vi "0630_Cinemática.vi"() -> ()   [LabVIEW 2017]
uses:
  <vilib>/robotics/Kinematics/Link/Joint Type.ctl
  <vilib>/robotics/Kinematics/RotateX.vi
  <vilib>/robotics/Kinematics/RotateY.vi
  <vilib>/robotics/Kinematics/RotateZ.vi
  <vilib>/Analysis/baseanly.llb/A x B.vi
  <vilib>/Analysis/baseanly.llb/Real A x B.vi
  <vilib>/robotics/Kinematics/Analytical/Initialize Generic Serial Arm.vi
  <vilib>/robotics/Kinematics/Robot/Inverse Kinematics (Point).vi
  <vilib>/picture/3D Picture Control/Object/Add Object (reference).vi
  <vilib>/robotics/Kinematics/Plotting/NI_Robotics_3DKinematics.lvlib
  <vilib>/robotics/Kinematics/Robot/NI_Robotics_Serial Robot Arm.lvclass
  <vilib>/robotics/Kinematics/Link/NI_Robotics_Link.lvclass
  <vilib>/robotics/Kinematics/Analytical/NI_Robotics_AnalyticKinematics.lvlib
  <vilib>/picture/3D Picture Control/NI_3D Picture Control.lvlib
  <vilib>/robotics/Kinematics/NI_Kinematics.lvlib
panel:
  in  "angles":cluster{"roll":dbl, "pitch":dbl, "yaw":dbl}
  in  "z":dbl
  in  "y":dbl
  in  "x":dbl
  out "error out":errorcluster
  out "3D Picture Control":refnum<vi>(3d-picture)
  in  "Stop Button":bool
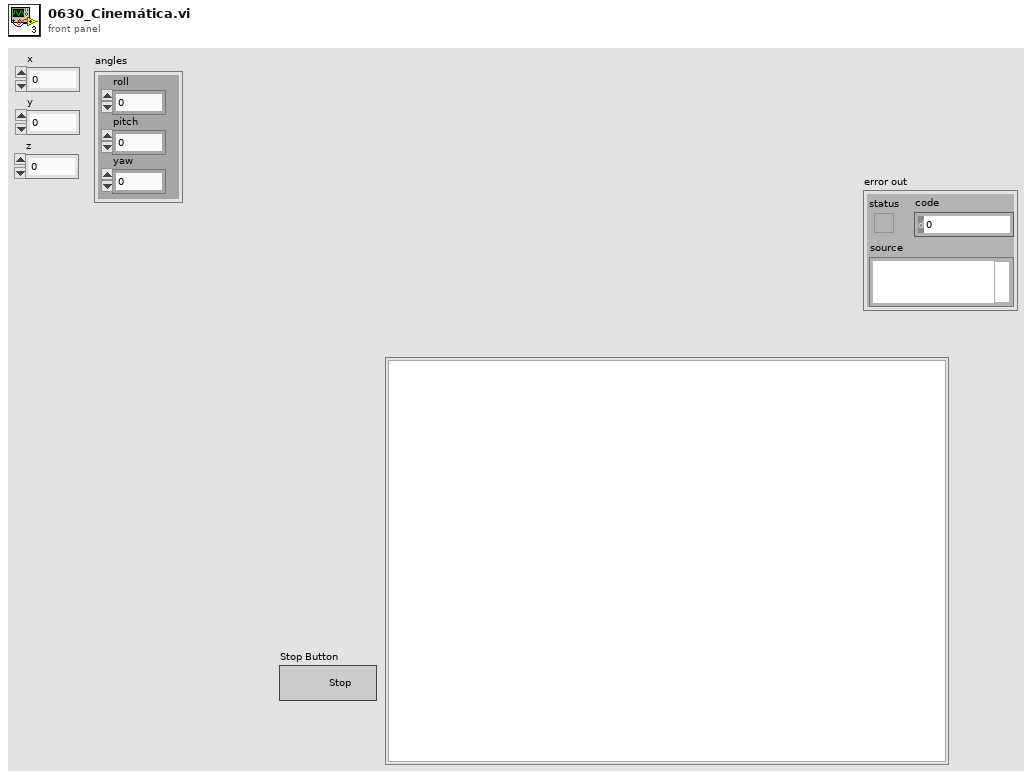
[diagram p1: front panel]
types:
  T1 = typedef "NI_Robotics_Link.lvclass/Joint Type.ctl" = enum16{"Revolute", "Prismatic"}
  T2 = cluster{"Twist Angle":dbl, "Length":dbl, "Rotation Angle":dbl, "Offset Distance":dbl, "Joint Type":T1, "Joint Coordinate Offset":dbl}[]
  T3 = typedef "NI_Matrix.lvlib/RealMatrix.ctl" = dbl[][]
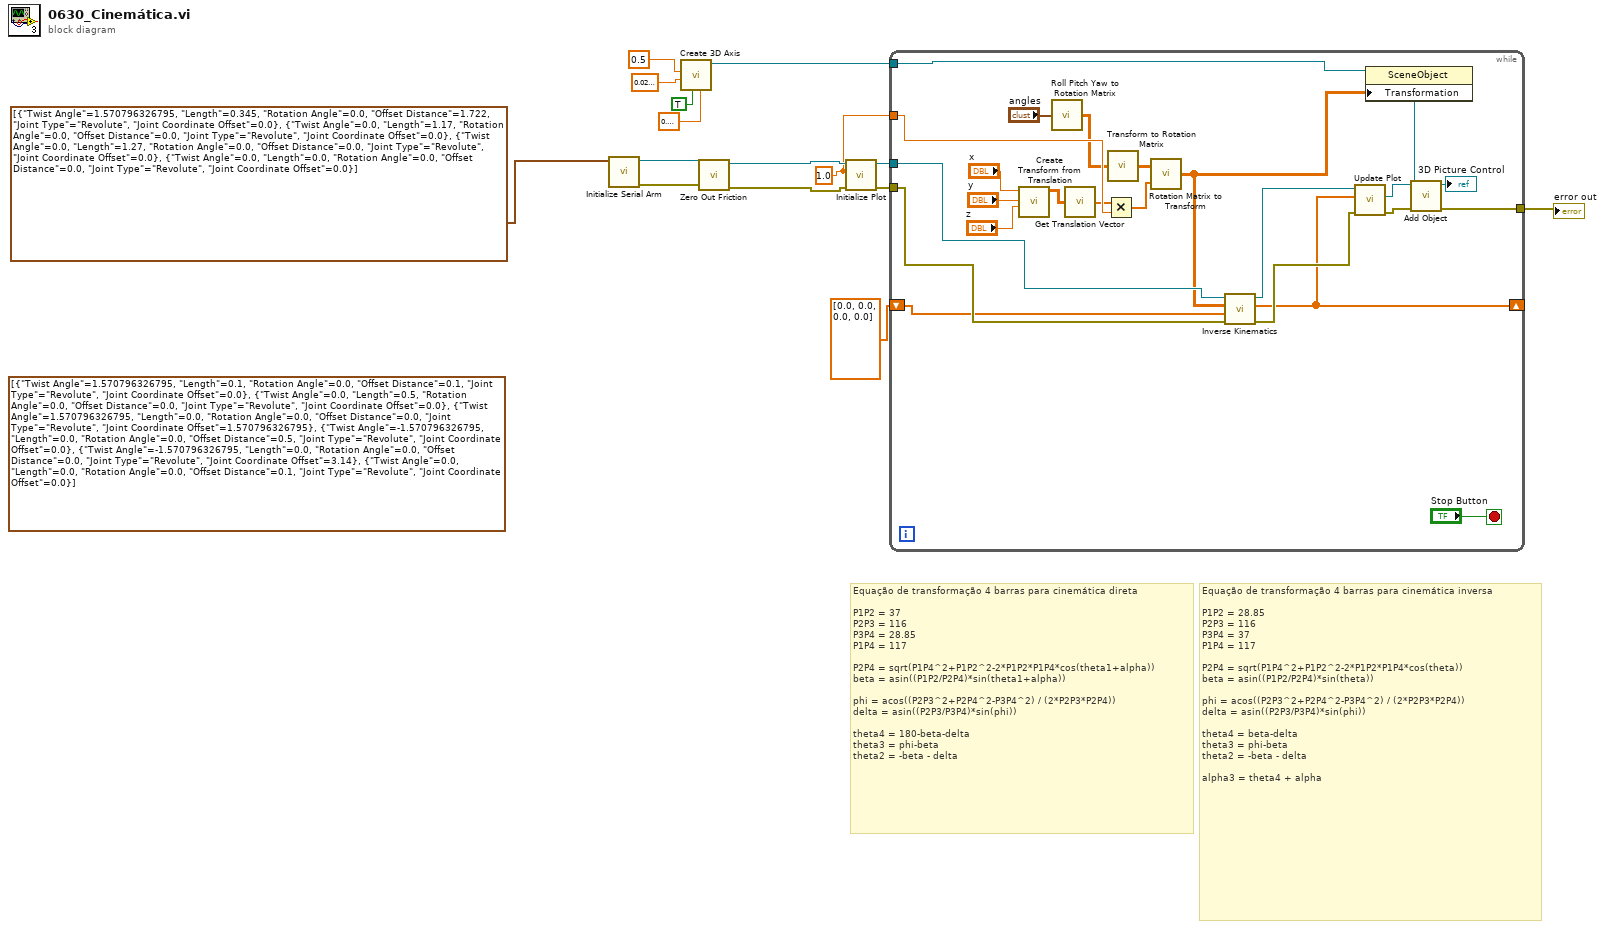
[diagram p0: block diagram]
diagram:
  (unwired) T2 [{"Twist Angle"=1.570796326795, "Length"=0.1, "Rotation Angle"=0.0, "Offset Distance"=0.1, "Joint Type"=enum."Revolute", "Joint Coordinate Offset"=0.0}, {"Twist Angle"=0.0, "Length"=0.5, "Rotation Angle"=0.0, "Offset Distance"=0.0, "Joint Type"=enum."Revolute", "Joint Coordinate Offset"=0.0}, {"Twist Angle"=1.570796326795, "Length"=0.0, "Rotation Angle"=0.0, "Offset Distance"=0.0, "Joint Type"=enum."Revolute", "Joint Coordinate Offset"=1.570796326795}, {"Twist Angle"=-1.570796326795, "Length"=0.0, "Rotation Angle"=0.0, "Offset Distance"=0.5, "Joint Type"=enum."Revolute", "Joint Coordinate Offset"=0.0}, {"Twist Angle"=-1.570796326795, "Length"=0.0, "Rotation Angle"=0.0, "Offset Distance"=0.0, "Joint Type"=enum."Revolute", "Joint Coordinate Offset"=3.14}, {"Twist Angle"=0.0, "Length"=0.0, "Rotation Angle"=0.0, "Offset Distance"=0.1, "Joint Type"=enum."Revolute", "Joint Coordinate Offset"=0.0}]
  w4 = 1.0 ("scale (1)")
  # "Equação de transformação 4 barras para cinemática inversa\n\nP1P2 = 28.85\nP2P3 = 116\nP3P4 = 37\nP1P4 = 117\n\nP2P4 = sqrt(P1P4^2+P1P2^2-2*P1P2*P1P4*cos(theta))\nbeta = asin((P1P2/P2P4)*sin(theta))\n\nphi = acos((P2P3^2+P2P4^2-P3P4^2) / (2*P2P3*P2P4))\ndelta = asin((P2P3/P3P4)*sin(phi))\n\ntheta4 = beta-delta\ntheta3 = phi-beta\ntheta2 = -beta - delta\n\nalpha3 = theta4 + alpha"
  # "Equação de transformação 4 barras para cinemática direta\n\nP1P2 = 37\nP2P3 = 116\nP3P4 = 28.85\nP1P4 = 117\n\nP2P4 = sqrt(P1P4^2+P1P2^2-2*P1P2*P1P4*cos(theta1+alpha))\nbeta = asin((P1P2/P2P4)*sin(theta1+alpha))\n\nphi = acos((P2P3^2+P2P4^2-P3P4^2) / (2*P2P3*P2P4))\ndelta = asin((P2P3/P3P4)*sin(phi))\n\ntheta4 = 180-beta-delta\ntheta3 = phi-beta\ntheta2 = -beta - delta"
  n1 = call-poly <vilib>:"Initialize Serial Arm.vi"("kinematic parameters"=T2 [{"Twist Angle"=1.570796326795, "Length"=0.345, "Rotation Angle"=0.0, "Offset Distance"=1.722, "Joint Type"=enum."Revolute", "Joint Coordinate Offset"=0.0}, {"Twist Angle"=0.0, "Length"=1.17, "Rotation Angle"=0.0, "Offset Distance"=0.0, "Joint Type"=enum."Revolute", "Joint Coordinate Offset"=0.0}, {"Twist Angle"=0.0, "Length"=1.27, "Rotation Angle"=0.0, "Offset Distance"=0.0, "Joint Type"=enum."Revolute", "Joint Coordinate Offset"=0.0}, {"Twist Angle"=0.0, "Length"=0.0, "Rotation Angle"=0.0, "Offset Distance"=0.0, "Joint Type"=enum."Revolute", "Joint Coordinate Offset"=0.0}]) -> ("error out"=w10:errorcluster, "serial arm out"=w11:refnum<class "NI_Robotics_Serial Robot Arm.lvclass">)  [unwired: 9 in]
  n2 = call <vilib>:"Create 3D Axis.vi"("Character Size"=sgl 0.2, "Axis label?"=TRUE, "Radius"=sgl 0.03, "Length"=sgl 0.5) -> ("New Object Refnum"=w8:refnum<vi>)  [unwired: 6 in, 1 out]
  n3 = call <vilib>:"Zero Out Friction.vi"("error in (no error)"=w10, "serial arm in"=w11) -> ("error out"=w13:errorcluster, "serial arm out"=w14:refnum<class "NI_Robotics_Serial Robot Arm.lvclass">)  [unwired: 8 in]
  n4 = call <vilib>:"Initialize Plot.vi"("error in (no error)"=w13, "scale (1)"=w4, "serial arm in"=w14) -> ("error out"=w12:errorcluster, "serial arm out"=w15:refnum<class "NI_Robotics_Serial Robot Arm.lvclass">)  [unwired: 7 in]
  n5 = while {
    tunnel: w15 -> [w27]
    tunnel: w12 -> [w26]
    tunnel: w8 -> [w37]
    tunnel: w4 -> [w33]
    tunnel: [w32] -> w2
    shift-right: [w19] -> _
    shift-left: dbl[] [0.0, 0.0, 0.0, 0.0] ("joint positions") -> [w18]
    stop <- "Stop Button" stop-if-true
    n6 = call <vilib>:"Create Transform from Translation.vi"("z"="z", "y"="y", "x"="x") -> ("transform"=w24:T3)  [unwired: 8 in]
    n7 = call <vilib>:"Roll Pitch Yaw to Rotation Matrix.vi"("angles"="angles") -> ("rotation matrix"=w17:T3)
    n8 = call <vilib>:"Get Translation Vector.vi"("transform"=w24) -> ("translation vector"=w30:dbl[])
    n9 = Multiply(x=w30, y=w33) -> (x*y=w31:dbl[])
    n10 = call <vilib>:"Transform to Rotation Matrix.vi"("transform"=w17) -> ("rotation matrix"=w29:T3)
    n11 = call <vilib>:"Rotation Matrix to Transform.vi"("translation vector"=w31, "rotation matrix"=w29) -> ("transform"=w20:T3)
    n12 = call-poly <vilib>:"Inverse Kinematics.vi"("error in (no error)"=w26, "current joint positions"=w18, "end effector transform"=w20, "serial arm in"=w27) -> ("error out"=w25:errorcluster, "joint positions"=w19:dbl[], "serial arm out"=w28:refnum<class "NI_Robotics_Serial Robot Arm.lvclass">)  [unwired: 4 in, 1 out]
    n13 = call <vilib>:"Update Plot.vi"("error in (no error)"=w25, "joint positions"=w19, "serial arm in"=w28) -> ("error out"=w35:errorcluster, "serial arm scene"=w38:refnum<vi>)  [unwired: 6 in, 1 out]
    n14 = property class="SceneObject"(reference=w37, "Transformation"=w20) -> (reference out=w34:refnum<vi>)  [unwired: 1 in, 1 out]
    n15 = call-poly <vilib>:"Add Object.vi"("error in (no error)"=w35, "New Object In"=w34, "Scene Object In"=w38) -> ("error out"=w32:errorcluster, "Scene Object Out"=→"3D Picture Control":refnum<vi>)  [unwired: 6 in, 1 out]
  }
  "error out" <- w2
